vi "FGV_CriticalOpalescenceControl.vi"(7 "CO Actions":T1, 8 "Error In":errorcluster, 9 "Value":i32, 11 "VISA Refnum in":refnum<visa-resource-name>="COM1") -> (0 "Error Out":errorcluster, 1 "read buffer":string, 3 "VISA Refnum out":refnum<visa-resource-name>="COM1")   [LabVIEW 2014]
uses:
  Typedef_CriticalOpalescence_Actions.ctl
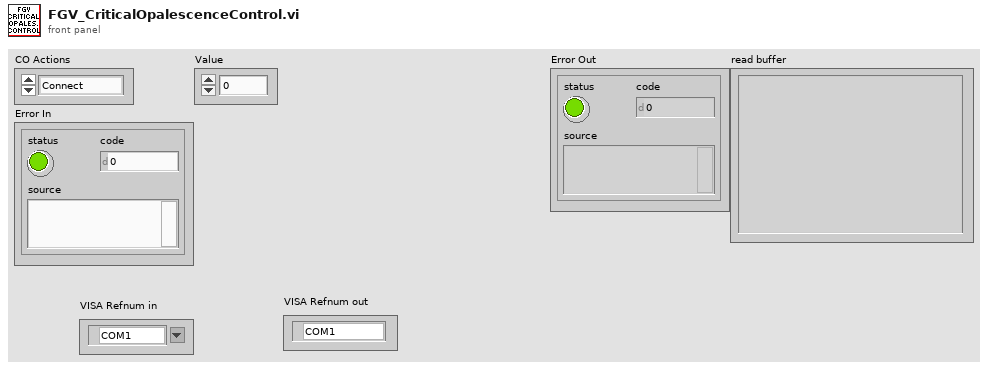
[diagram p1: front panel]
types:
  T1 = typedef "Typedef_CriticalOpalescence_Actions.ctl" = enum16{"Connect", "Disconnect", "Get Reading", "Set Coarse CoeffA", "Set Coarse CoeffB", "Set Fine CoeffA", "Set Fine CoeffB", "Set PD CoeffA", "Set PD CoeffB", "Get Coarse CoeffA", "Get Coarse CoeffB", "Get Fine CoeffA", "Get Fine CoeffB", "Get PD CoeffA", "Get PD CoeffB", "Set Time Step", "Get Time Step", "Save Settings", "Disable Readings", "Enable Readings"}
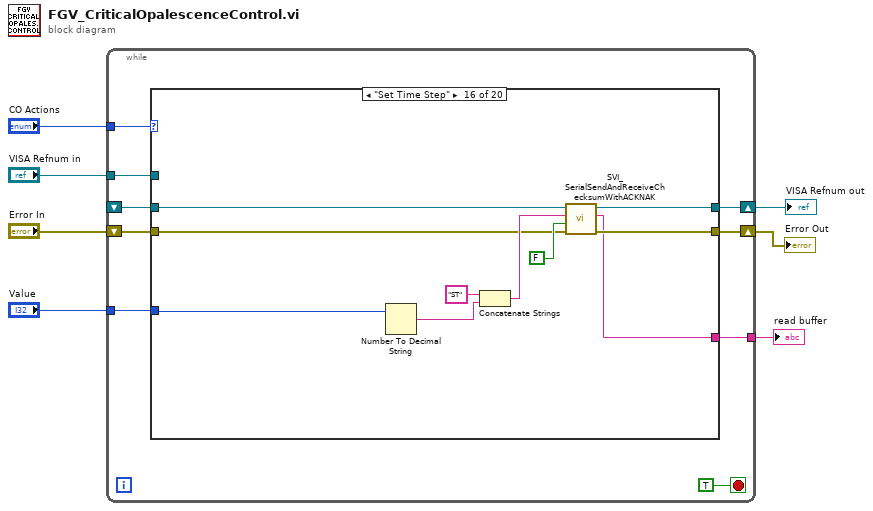
[diagram p0: block diagram]
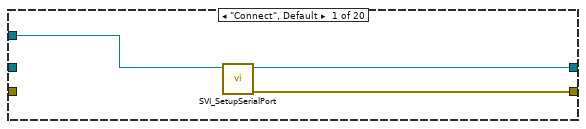
[diagram p2: hidden frame]
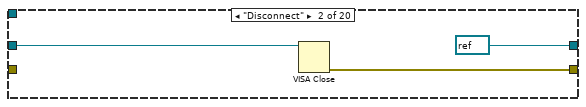
[diagram p3: hidden frame]
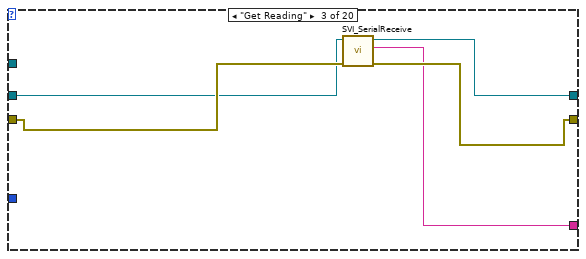
[diagram p4: hidden frame]
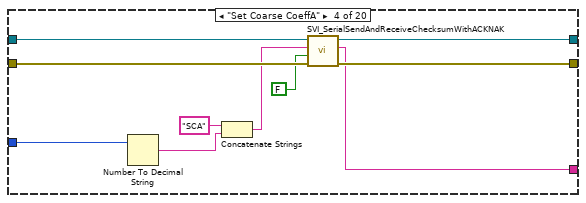
[diagram p5: hidden frame]
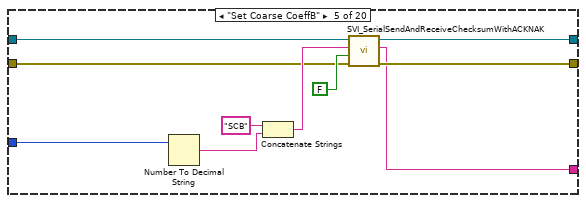
[diagram p6: hidden frame]
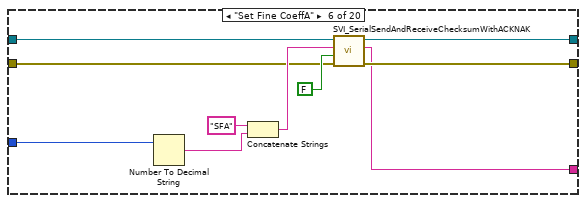
[diagram p7: hidden frame]
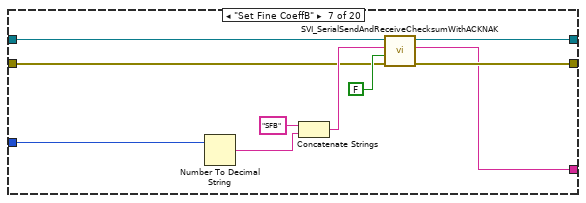
[diagram p8: hidden frame]
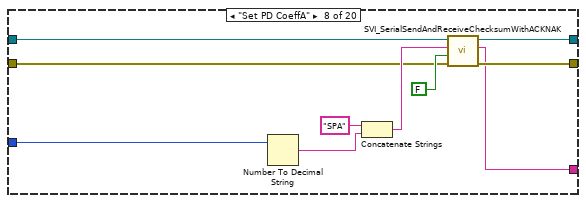
[diagram p9: hidden frame]
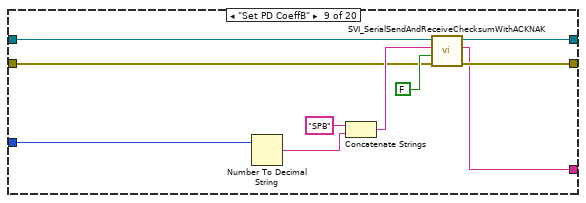
[diagram p10: hidden frame]
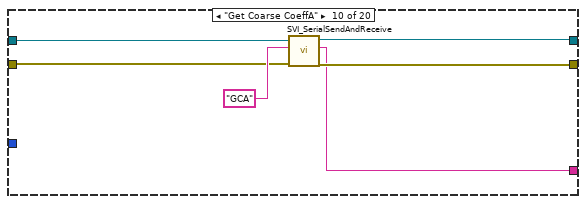
[diagram p11: hidden frame]
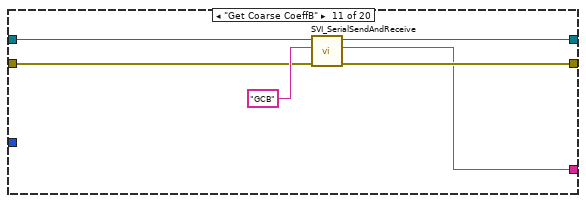
[diagram p12: hidden frame]
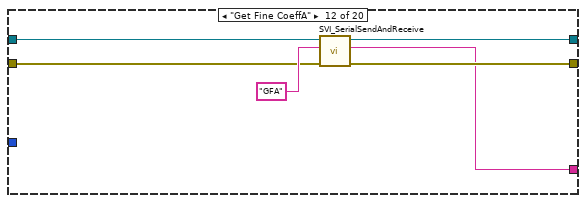
[diagram p13: hidden frame]
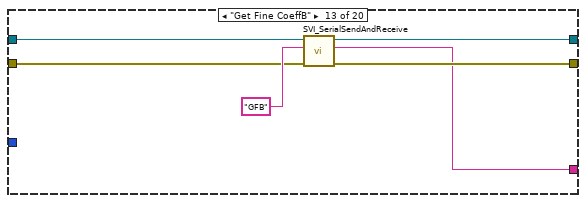
[diagram p14: hidden frame]
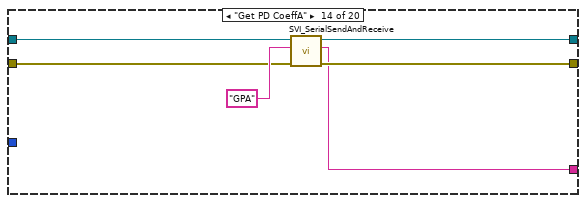
[diagram p15: hidden frame]
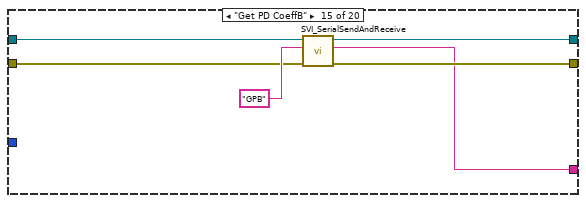
[diagram p16: hidden frame]
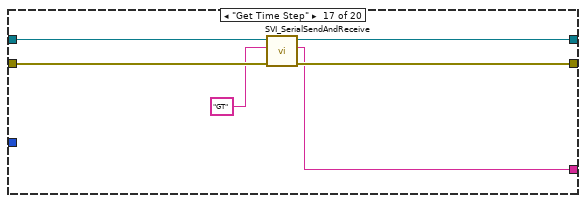
[diagram p17: hidden frame]
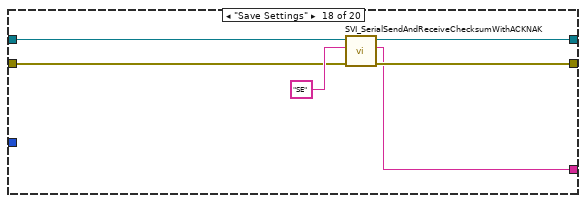
[diagram p18: hidden frame]
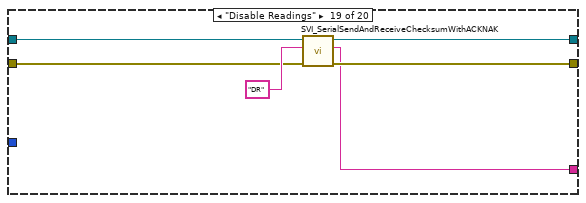
[diagram p19: hidden frame]
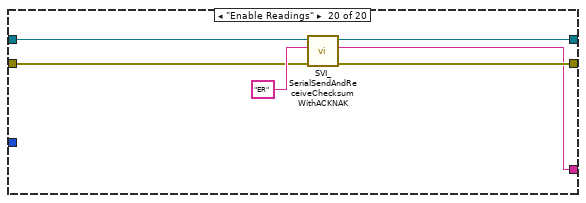
[diagram p20: hidden frame]
diagram:
  n1 = while {
    tunnel: "CO Actions" -> [w15]
    tunnel: "VISA Refnum in" -> [w14]
    shift-right: [w13] -> w3
    shift-left: _ -> [w11]
    shift-right: [w12] -> w5
    shift-left: "Error In" -> [w10]
    tunnel: "Value" -> [w9]
    tunnel: [w8] -> w1
    stop <- TRUE stop-if-true
    n2 = case shown="\"Set Time Step\"" w15 {
      tunnel: w14 -> [w19 _ _ _ _ _ _ _ _ _ _ _ _ _ _ _ _ _ _ _]
      tunnel: [w18 refnum<visa-resource-name> refnum ("VISA resource name out") w24 w33 w42 w53 w60 w70 w79 w90 w97 w102 w109 w115 w121 w126 w138 w143 w148 w154] -> w13
      tunnel: [w17 w22 w25 w34 w43 w52 w61 w71 w80 w89 w98 w103 w110 w116 w122 w127 w139 w144 w147 w153] -> w12
      tunnel: w11 -> [_ w20 w26 w36 w39 w50 w62 w72 w82 w91 w94 w100 w106 w114 w118 w128 w136 w142 w149 w155]
      tunnel: w10 -> [_ _ w27 w35 w40 w51 w63 w73 w83 w92 w95 w104 w107 w113 w119 w129 w137 w141 w150 w156]
      tunnel: w9 -> [_ _ _ w31 w38 w49 w58 w68 w81 _ _ _ _ _ _ w125 _ _ _ _]
      tunnel: [_ _ w23 w28 w41 w48 w59 w69 w78 w88 w96 w101 w108 w112 w120 w124 w134 w140 w146 w152] -> w8
      frame "Connect", Default {
        n3 = call "SVI_SetupSerialPort.vi"("VISA Refnum in"=w19) -> ("error out"=w17:errorcluster, "VISA Refnum out"=w18:refnum<visa-resource-name>)  [unwired: 9 in]
      }
      frame "Disconnect" {
        n4 = VISA Close(VISA resource name=w20) -> (error out=w22:errorcluster)  [unwired: 1 in]
      }
      frame "Get Reading" {
        n5 = call "SVI_SerialReceive.vi"("error in (no error)"=w27, "VISA Refnum in"=w26) -> ("error out"=w25:errorcluster, "read buffer"=w23:string, "VISA resource name out"=w24:refnum<visa-resource-name>)  [unwired: 7 in]
      }
      frame "Set Coarse CoeffA" {
        n6 = Number To Decimal String(number=w31) -> (decimal integer string=w29:string)  [unwired: 1 in]
        n7 = Concatenate Strings("SCA" ("Command"), w29) -> (w30:string)
        n8 = call "SVI_SerialSendAndReceiveChecksumWithACKNAK.vi"("error in (no error)"=w35, "Send Checksum"=FALSE, "Command"=w30, "VISA Refnum in"=w36) -> ("error out"=w34:errorcluster, "Received"=w28:string, "VISA resource name out"=w33:refnum<visa-resource-name>)  [unwired: 5 in]
      }
      frame "Set Coarse CoeffB" {
        n9 = Number To Decimal String(number=w38) -> (decimal integer string=w44:string)  [unwired: 1 in]
        n10 = Concatenate Strings("SCB" ("Command"), w44) -> (w45:string)
        n11 = call "SVI_SerialSendAndReceiveChecksumWithACKNAK.vi"("error in (no error)"=w40, "Send Checksum"=FALSE, "Command"=w45, "VISA Refnum in"=w39) -> ("error out"=w43:errorcluster, "Received"=w41:string, "VISA resource name out"=w42:refnum<visa-resource-name>)  [unwired: 5 in]
      }
      frame "Set Fine CoeffA" {
        n12 = Number To Decimal String(number=w49) -> (decimal integer string=w54:string)  [unwired: 1 in]
        n13 = Concatenate Strings("SFA" ("Command"), w54) -> (w55:string)
        n14 = call "SVI_SerialSendAndReceiveChecksumWithACKNAK.vi"("error in (no error)"=w51, "Send Checksum"=FALSE, "Command"=w55, "VISA Refnum in"=w50) -> ("error out"=w52:errorcluster, "Received"=w48:string, "VISA resource name out"=w53:refnum<visa-resource-name>)  [unwired: 5 in]
      }
      frame "Set Fine CoeffB" {
        n15 = Number To Decimal String(number=w58) -> (decimal integer string=w64:string)  [unwired: 1 in]
        n16 = Concatenate Strings("SFB" ("Command"), w64) -> (w65:string)
        n17 = call "SVI_SerialSendAndReceiveChecksumWithACKNAK.vi"("error in (no error)"=w63, "Send Checksum"=FALSE, "Command"=w65, "VISA Refnum in"=w62) -> ("error out"=w61:errorcluster, "Received"=w59:string, "VISA resource name out"=w60:refnum<visa-resource-name>)  [unwired: 5 in]
      }
      frame "Set PD CoeffA" {
        n18 = Number To Decimal String(number=w68) -> (decimal integer string=w74:string)  [unwired: 1 in]
        n19 = Concatenate Strings("SPA" ("Command"), w74) -> (w75:string)
        n20 = call "SVI_SerialSendAndReceiveChecksumWithACKNAK.vi"("error in (no error)"=w73, "Send Checksum"=FALSE, "Command"=w75, "VISA Refnum in"=w72) -> ("error out"=w71:errorcluster, "Received"=w69:string, "VISA resource name out"=w70:refnum<visa-resource-name>)  [unwired: 5 in]
      }
      frame "Set PD CoeffB" {
        n21 = Number To Decimal String(number=w81) -> (decimal integer string=w84:string)  [unwired: 1 in]
        n22 = Concatenate Strings("SPB" ("Command"), w84) -> (w85:string)
        n23 = call "SVI_SerialSendAndReceiveChecksumWithACKNAK.vi"("error in (no error)"=w83, "Send Checksum"=FALSE, "Command"=w85, "VISA Refnum in"=w82) -> ("error out"=w80:errorcluster, "Received"=w78:string, "VISA resource name out"=w79:refnum<visa-resource-name>)  [unwired: 5 in]
      }
      frame "Get Coarse CoeffA" {
        n24 = call "SVI_SerialSendAndReceive.vi"("error in (no error)"=w92, "Command"="GCA", "VISA Refnum in"=w91) -> ("error out"=w89:errorcluster, "read buffer"=w88:string, "VISA resource name out"=w90:refnum<visa-resource-name>)  [unwired: 6 in]
      }
      frame "Get Coarse CoeffB" {
        n25 = call "SVI_SerialSendAndReceive.vi"("error in (no error)"=w95, "Command"="GCB", "VISA Refnum in"=w94) -> ("error out"=w98:errorcluster, "read buffer"=w96:string, "VISA resource name out"=w97:refnum<visa-resource-name>)  [unwired: 6 in]
      }
      frame "Get Fine CoeffA" {
        n26 = call "SVI_SerialSendAndReceive.vi"("error in (no error)"=w104, "Command"="GFA", "VISA Refnum in"=w100) -> ("error out"=w103:errorcluster, "read buffer"=w101:string, "VISA resource name out"=w102:refnum<visa-resource-name>)  [unwired: 6 in]
      }
      frame "Get Fine CoeffB" {
        n27 = call "SVI_SerialSendAndReceive.vi"("error in (no error)"=w107, "Command"="GFB", "VISA Refnum in"=w106) -> ("error out"=w110:errorcluster, "read buffer"=w108:string, "VISA resource name out"=w109:refnum<visa-resource-name>)  [unwired: 6 in]
      }
      frame "Get PD CoeffA" {
        n28 = call "SVI_SerialSendAndReceive.vi"("error in (no error)"=w113, "Command"="GPA", "VISA Refnum in"=w114) -> ("error out"=w116:errorcluster, "read buffer"=w112:string, "VISA resource name out"=w115:refnum<visa-resource-name>)  [unwired: 6 in]
      }
      frame "Get PD CoeffB" {
        n29 = call "SVI_SerialSendAndReceive.vi"("error in (no error)"=w119, "Command"="GPB", "VISA Refnum in"=w118) -> ("error out"=w122:errorcluster, "read buffer"=w120:string, "VISA resource name out"=w121:refnum<visa-resource-name>)  [unwired: 6 in]
      }
      frame "Set Time Step" {
        n30 = Number To Decimal String(number=w125) -> (decimal integer string=w130:string)  [unwired: 1 in]
        n31 = Concatenate Strings("ST" ("Command"), w130) -> (w131:string)
        n32 = call "SVI_SerialSendAndReceiveChecksumWithACKNAK.vi"("error in (no error)"=w129, "Send Checksum"=FALSE, "Command"=w131, "VISA Refnum in"=w128) -> ("error out"=w127:errorcluster, "Received"=w124:string, "VISA resource name out"=w126:refnum<visa-resource-name>)  [unwired: 5 in]
      }
      frame "Get Time Step" {
        n33 = call "SVI_SerialSendAndReceive.vi"("error in (no error)"=w137, "Command"="GT", "VISA Refnum in"=w136) -> ("error out"=w139:errorcluster, "read buffer"=w134:string, "VISA resource name out"=w138:refnum<visa-resource-name>)  [unwired: 6 in]
      }
      frame "Save Settings" {
        n34 = call "SVI_SerialSendAndReceiveChecksumWithACKNAK.vi"("error in (no error)"=w141, "Command"="SE", "VISA Refnum in"=w142) -> ("error out"=w144:errorcluster, "Received"=w140:string, "VISA resource name out"=w143:refnum<visa-resource-name>)  [unwired: 6 in]
      }
      frame "Disable Readings" {
        n35 = call "SVI_SerialSendAndReceiveChecksumWithACKNAK.vi"("error in (no error)"=w150, "Command"="DR", "VISA Refnum in"=w149) -> ("error out"=w147:errorcluster, "Received"=w146:string, "VISA resource name out"=w148:refnum<visa-resource-name>)  [unwired: 6 in]
      }
      frame "Enable Readings" {
        n36 = call "SVI_SerialSendAndReceiveChecksumWithACKNAK.vi"("error in (no error)"=w156, "Command"="ER", "VISA Refnum in"=w155) -> ("error out"=w153:errorcluster, "Received"=w152:string, "VISA resource name out"=w154:refnum<visa-resource-name>)  [unwired: 6 in]
      }
    }
  }
  "VISA Refnum out" <- w3
  "Error Out" <- w5
  "read buffer" <- w1
